vi "Install CDF.vi"(6 "Target Config":T3={"IP Address"="0.0.0.0", "Target"=enum."cRIO-9012", "Username"="", "Password"=""}, 8 "error in (no error)":errorcluster, 10 "Sys Cfg Session In":refnum<k21>, 11 "Console Ref In":refnum<vi>) -> (0 "error out":errorcluster, 2 "Sys Cfg Session Out":refnum<k21>, 3 "Console Ref Out":refnum<vi>)   [LabVIEW 2015]
doc: "Install the appropriate CDF file to the target dependent on it's operating system."
uses:
  Type Defs/Target Config Cluster.ctl
  Type Defs/RT Target Type.ctl
  <vilib>/nisyscfg/Software 1.2.ctl
  <vilib>/nisyscfg/Component Type.ctl
  <vilib>/nisyscfg/Get Available Components.vi
  <vilib>/nisyscfg/Install or Uninstall Components.vi
  <vilib>/nisyscfg/nisyscfg.lvlib
panel:
  out "software components":T1[](array[typedef]) {"component type" items=["standard", "hidden", "system", "unknown", "startup"]}
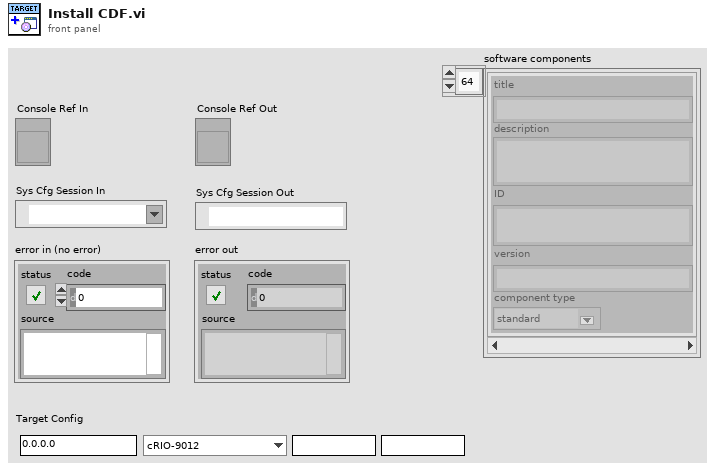
[diagram p1: front panel]
types:
  T1 = typedef "nisyscfg.lvlib/Software 1.2.ctl" = cluster{"title":string, "description":string, "ID":string, "version":string, "component type":T2}
  T2 = typedef "nisyscfg.lvlib/Component Type.ctl" = u32
  T3 = typedef "Target Config Cluster.ctl" = cluster{"IP Address":string, "Target":T4, "Username":string, "Password":string}
  T4 = typedef "RT Target Type.ctl" = enum16{"cRIO-9012", "cRIO-9014", "cRIO-9022", "cRIO-9023", "cRIO-9024", "cRIO-9025", "cRIO-9068", "cRIO-9073", "cRIO-9074", "cRIO-9075", "cRIO-9076", "cRIO-9081", "cRIO-9082", "myRIO-1900", "myRIO-1950", "PXI-8101", "PXI-8115", "PXI-8119", "PXI-8820", "PXIe-8100", "PXIe-8101", "PXIe-8133", "PXIe-8135", "PXIe-8820", "sbRIO-9605", "sbRIO-9606", "sbRIO-9623", "sbRIO-9626", "sbRIO-9633", "sbRIO-9636", "Unlisted (Linux-RT)", "Unlisted (PharLap)", "Unlisted (VxWorks)"}
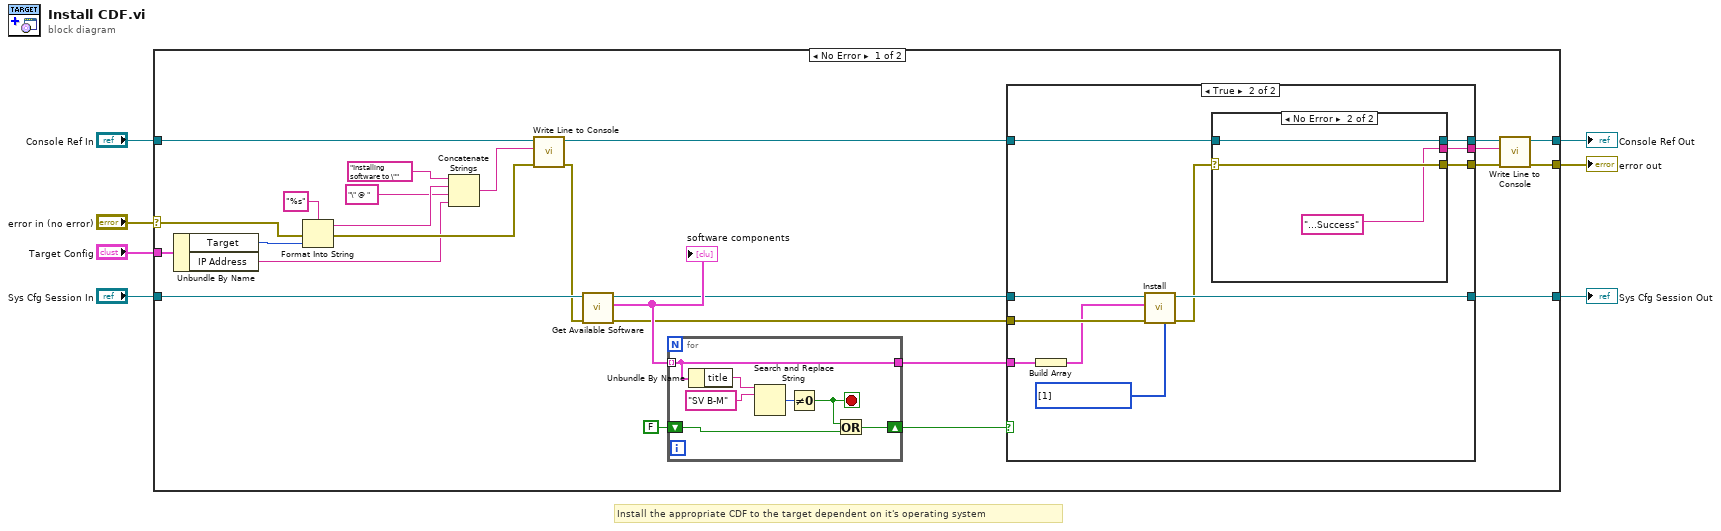
[diagram p0: block diagram]
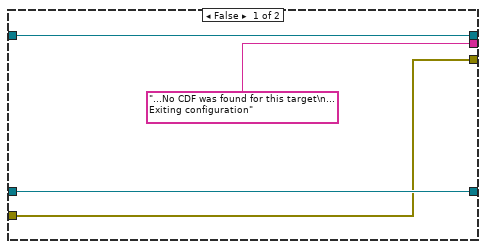
[diagram p2: hidden frame]
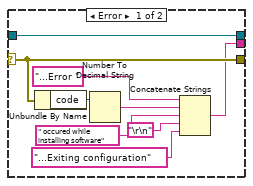
[diagram p3: hidden frame]
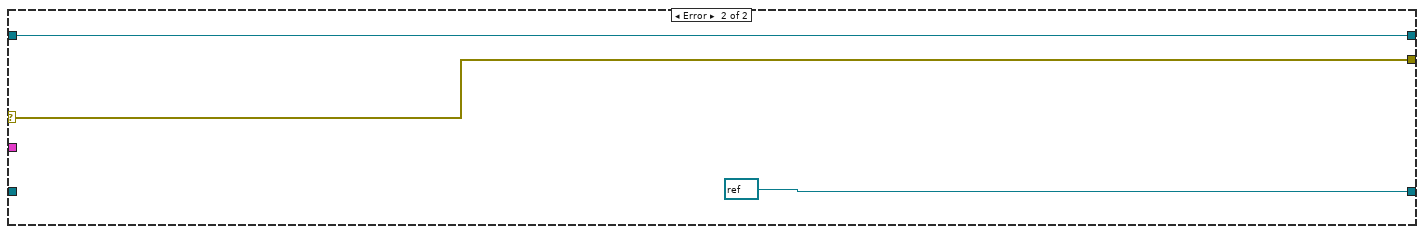
[diagram p4: hidden frame]
diagram:
  # "Install the appropriate CDF to the target dependent on it's operating system"
  n1 = case shown="No Error" "error in (no error)" {
    selector: "error in (no error)" -> [w31 w69]
    tunnel: "Console Ref In" -> [w27 w70]
    tunnel: "Target Config" -> [w33 _]
    tunnel: [w9 w70] -> w4
    tunnel: [w8 w69] -> w3
    tunnel: [w13 refnum<k21> refnum ("session out")] -> w2
    tunnel: "Sys Cfg Session In" -> [w24 _]
    frame No Error {
      n2 = Unbundle By Name(w33) -> ("Target"=w21:T4, "IP Address"=w22:string)
      n3 = Format Into String(format string="%s", error in=w31, w21) -> (resulting string=w29:string, error out=w26:errorcluster)  [unwired: 1 in]
      n4 = Concatenate Strings("Installing software to \"", w29, "\" @ ", w22) -> (w25:string)
      n5 = call "Write Line to Console.vi"("error in (no error)"=w26, "Line to Write"=w25, "Console Ref In"=w27) -> ("error out (no error)"=w23:errorcluster, "Console Ref In Out"=w18:refnum<vi>)  [unwired: 7 in]
      n6 = call-poly <vilib>:"Get Available Software.vi"("error in (no error)"=w23, "Session in"=w24) -> ("error out"=w15:errorcluster, "Software Components"=w20:T1[], "Session out"=w14:refnum<k21>)  [unwired: 7 in]
      "software components" <- w20
      n7 = for {
        tunnel: w20 -> [w67] mode=indexing
        tunnel: [w67] -> w16
        shift-right: [w66] -> w17
        shift-left: FALSE -> [w65]
        stop <- w62 stop-if-true
        n8 = Unbundle By Name(w67) -> ("title"=w64:string)
        n9 = Search and Replace String(input string=w64, search string="SV B-M" ("replace string (\"\")")) -> (number of replacements=w63:i32)  [unwired: 6 in, 3 out]
        n10 = Not Equal To 0?(x=w63) -> (x != 0?=w62:bool)
        n11 = Or(x=w62, y=w65) -> (x .or. y?=w66:bool)
      }
      n12 = case shown="True" w17 {
        tunnel: w18 -> [w37 w42]
        tunnel: w16 -> [_ w48]
        tunnel: w15 -> [w34 w47]
        tunnel: w14 -> [w36 w44]
        tunnel: [w36 w43] -> w13
        tunnel: [w37 w40] -> w12
        tunnel: ["...No CDF was found for this target\n...Exiting configuration" w39] -> w11
        tunnel: [w34 w38] -> w10
        frame False {
        }
        frame True {
          w45 = u32[] [1] items=["Highest", "Exactly"] ("version selection (highest)")
          n13 = Build Array(w48) -> (w46:T1[])
          n14 = call-poly <vilib>:"Install.vi"("Version Selection (Highest)"=w45, "error in (no error)"=w47, "Software Components to Install"=w46, "Session in"=w44) -> ("error out"=w41:errorcluster, "Session out"=w43:refnum<k21>)  [unwired: 5 in, 1 out]
          n15 = case shown="No Error" w41 {
            selector: w41 -> [w57 w60]
            tunnel: [w57 w60] -> w38
            tunnel: [w50 "...Success"] -> w39
            tunnel: [w49 w58] -> w40
            tunnel: w42 -> [w49 w58]
            frame Error {
              n16 = Unbundle By Name(w57) -> ("code"=w56:i32)
              n17 = Number To Decimal String(number=w56) -> (decimal integer string=w55:string)  [unwired: 1 in]
              n18 = Concatenate Strings("...Error ", w55, " occured while installing software", "\r\n", "...Exiting configuration") -> (w50:string)
            }
            frame No Error {
            }
          }
        }
      }
      n19 = call "Write Line to Console.vi"("error in (no error)"=w10, "Line to Write"=w11, "Console Ref In"=w12) -> ("error out (no error)"=w8:errorcluster, "Console Ref In Out"=w9:refnum<vi>)  [unwired: 7 in]
    }
    frame Error {
    }
  }
  "error out" <- w3
  "Console Ref Out" <- w4
  "Sys Cfg Session Out" <- w2
